vi "Subtract XY (single).vi"(8 "error in (no error)":errorcluster, 9 "y":cluster{"X-array":dbl[], "Y-array":dbl[]}, 10 "x":cluster{"X-array":dbl[], "Y-array":dbl[]}, 11 "XY-data":cluster{"X-array":dbl[], "Y-array":dbl[]}) -> (0 "error out":errorcluster, 3 "XY-data out":cluster{"X-array":dbl[], "Y-array":dbl[]} {"Y-array" format="%.2p"; "X-array" format="%.2p"})   [LabVIEW 2019, in "xy_utilities.lvlib"]
doc: "Subtract <b>x</b>'s x array from the x array of <b>XY-data</b>\nSubtract <b>y</b>'s y array from the y array of <b>XY-data</b>\n\nWire data to the data input to determine the polymorphic instance to use or manually select the instance."
uses:
  xy_utilities.lvlib
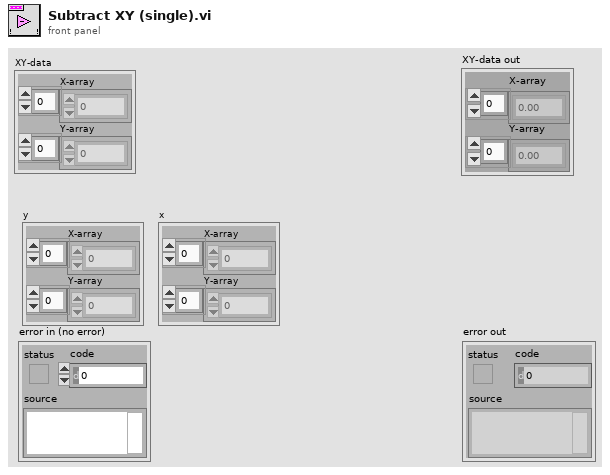
[diagram p1: front panel]
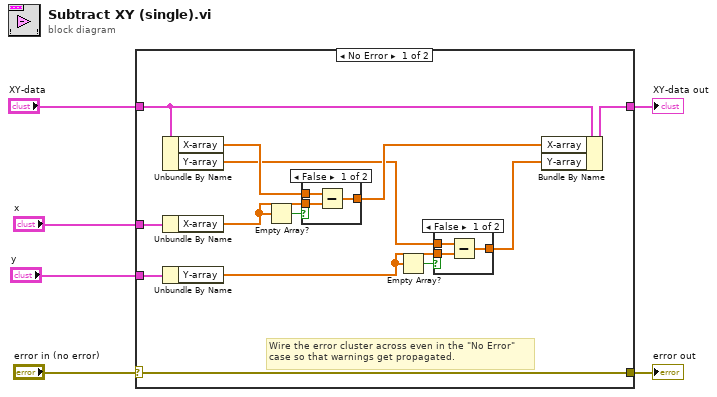
[diagram p0: block diagram]
diagram:
  n1 = case shown="No Error" "error in (no error)" {
    selector: "error in (no error)" -> [w19 w29]
    tunnel: [w19 w29] -> w5
    tunnel: "XY-data" -> [w18 w28]
    tunnel: [w17 w28] -> w3
    tunnel: "y" -> [w16 _]
    tunnel: "x" -> [w15 _]
    frame No Error {
      # "Wire the error cluster across even in the \"No Error\"\ncase so that warnings get propagated."
      n2 = Unbundle By Name(w18) -> ("X-array"=w11:dbl[], "Y-array"=w7:dbl[])
      n3 = Unbundle By Name(w15) -> ("X-array"=w10:dbl[])
      n4 = Unbundle By Name(w16) -> ("Y-array"=w12:dbl[])
      n5 = Empty Array?(array=w10) -> (empty?=w14:bool)
      n6 = case shown="False" w14 {
        tunnel: w10 -> [w22 _]
        tunnel: w11 -> [w21 w23]
        tunnel: [w20 w23] -> w8
        frame False {
          n7 = Subtract(x=w21, y=w22) -> (x-y=w20:dbl[])
        }
        frame True {
        }
      }
      n8 = Empty Array?(array=w12) -> (empty?=w13:bool)
      n9 = case shown="False" w13 {
        tunnel: w12 -> [w26 _]
        tunnel: w7 -> [w24 w27]
        tunnel: [w25 w27] -> w9
        frame False {
          n10 = Subtract(x=w24, y=w26) -> (x-y=w25:dbl[])
        }
        frame True {
        }
      }
      n11 = Bundle By Name(cluster=w18, "X-array"=w8, "Y-array"=w9) -> (w17:cluster{"X-array":dbl[], "Y-array":dbl[]})
    }
    frame Error {
    }
  }
  "error out" <- w5
  "XY-data out" <- w3
